vi "19052 Get_PA_TIME.vi"(8 "error in (no error)":errorcluster, 9 "Step":u16=1 min=1 max=99 step=1, 11 "VISA resource in":refnum<visa-resource-name>) -> (0 "error out":errorcluster, 1 "Pause Time":dbl format="%.1p", 3 "VISA resource out":refnum<visa-resource-name>)   [LabVIEW 2015]
panel:
  out "output command":string
  # "Get PA TIME"
  # "0.3 <= time <= 999.0\n0 = CONT."
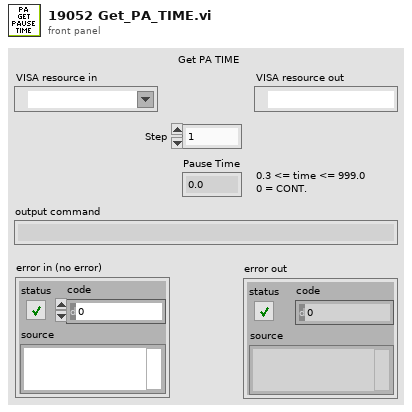
[diagram p1: front panel]
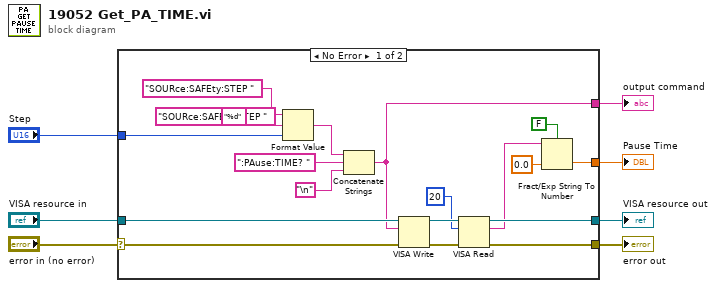
[diagram p0: block diagram]
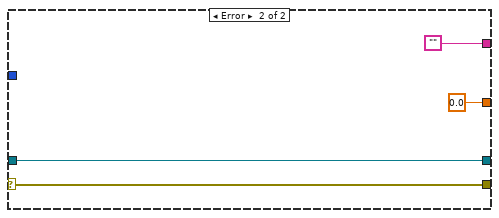
[diagram p2: hidden frame]
diagram:
  n1 = case shown="No Error" "error in (no error)" {
    selector: "error in (no error)" -> [w25 w29]
    tunnel: [w13 w29] -> w7
    tunnel: "Step" -> [w23 _]
    tunnel: [w20 ""] -> w4
    tunnel: [w14 w28] -> w3
    tunnel: "VISA resource in" -> [w21 w28]
    tunnel: [w9 0.0] -> w1
    frame No Error {
      (unwired) "SOURce:SAFEty:STEP "
      n2 = Format Value(string ("")="SOURce:SAFEty:STEP ", format string="%d", value (0)=w23) -> (output string=w18:string)
      n3 = Concatenate Strings(w18, ":PAuse:TIME? ", "\n") -> (w20:string)
      n4 = VISA Write(VISA resource name=w21, write buffer=w20, error in (no error)=w25) -> (VISA resource name out=w15:refnum<visa-resource-name>, error out=w16:errorcluster)  [unwired: 1 out]
      n5 = VISA Read(VISA resource name=w15, byte count=u32 20, error in (no error)=w16) -> (VISA resource name out=w14:refnum<visa-resource-name>, read buffer=w10:string, error out=w13:errorcluster)  [unwired: 1 out]
      n6 = Fract/Exp String To Number(use system decimal point (T)=FALSE, string=w10, default (0 dbl)=0.0 ("default (0 DBL)")) -> (number=w9:dbl)  [unwired: 1 in, 1 out]
    }
    frame Error {
    }
  }
  "error out" <- w7
  "output command" <- w4
  "VISA resource out" <- w3
  "Pause Time" <- w1
